vi "Manual Post Build.vi"() -> ()   [LabVIEW 2019]
uses:
  <userlib>/LevyLab/Build Support/PostBuildSupport/PostBuildSupport.lvclass
panel:
  out "error out":errorcluster
  in  "Output Package File Path":path=path "C:/user/patrick/git/Multichannel-Lockin/builds/Package"
  in  "Product Name":string="Multichannel Lockin"
  in  "Package Version":string="2.8.9.18"
  in  "Package Source Folder":path=path "C:/user/patrick/git/Multichannel-Lockin/src"
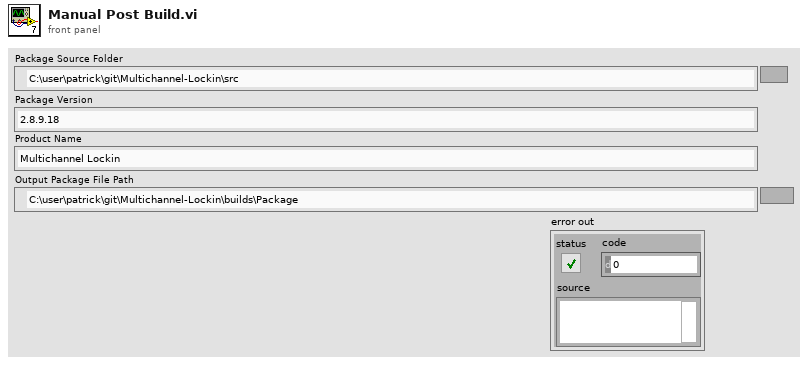
[diagram p1: front panel]
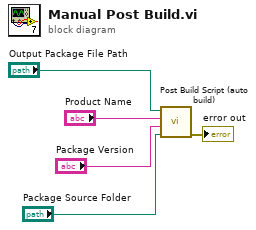
[diagram p0: block diagram]
diagram:
  n1 = call <userlib>:"Post Build Script (auto build).vi"("Package Source Folder"="Package Source Folder", "Package Version"="Package Version", "Product Name"="Product Name", "Output Package File Path"="Output Package File Path") -> ("error out"=→"error out":errorcluster)  [unwired: 7 in]
